vi "ReadGatewayConfigurationFile.vi"(8 "error in (no error)":errorcluster, 11 "targets.ini file":path) -> (0 "error out":errorcluster, 3 "Gateway Configuration":T1)   [LabVIEW 2024, in "VeriStandTestUtilities.lvlib"]
uses:
  VeriStandTestUtilities.lvlib
  GatewayConfiguration.ctl
  <vilib>/Utility/config.llb/Read Key (String).vi
  <vilib>/Utility/config.llb/NI_LVConfig.lvlib
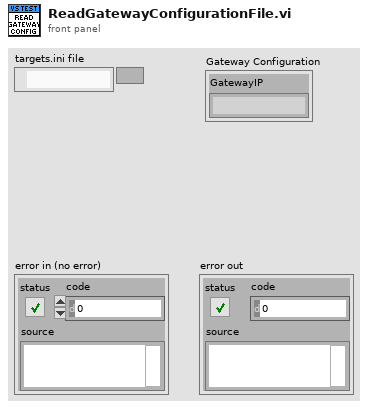
[diagram p1: front panel]
types:
  T1 = typedef "VeriStandTestUtilities.lvlib/GatewayConfiguration.ctl" = cluster{"GatewayIP":string}
  T2 = typedef "NI_LVConfig.lvlib/Config Data RefNum.ctl" = refnum<k1>
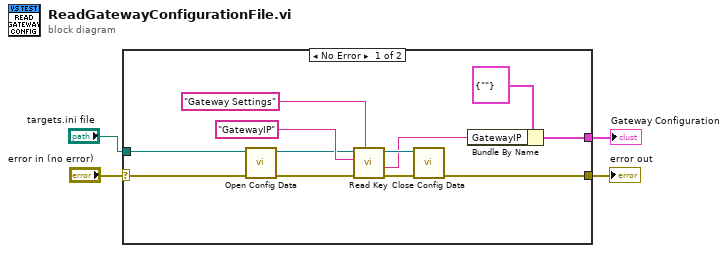
[diagram p0: block diagram]
diagram:
  n1 = case shown="No Error" "error in (no error)" {
    selector: "error in (no error)" -> [w15 w17]
    tunnel: [w6 w17] -> w3
    tunnel: "targets.ini file" -> [w16 _]
    tunnel: [w10 _] -> w1
    frame No Error {
      n2 = call <vilib>:"Open Config Data.vi"("error in (no error)"=w15, "configuration file path"=w16) -> ("error out"=w8:errorcluster, "refnum"=w9:T2)  [unwired: 7 in, 1 out]
      n3 = call-poly <vilib>:"Read Key.vi"("section"="Gateway Settings", "error in (no error)"=w8, "key"="GatewayIP", "refnum"=w9) -> ("error out"=w14:errorcluster, "value"=w5:string, "refnum out"=w13:T2)  [unwired: 4 in, 1 out]
      n4 = call <vilib>:"Close Config Data.vi"("error in (no error)"=w14, "refnum"=w13) -> ("error out"=w6:errorcluster)  [unwired: 8 in, 1 out]
      n5 = Bundle By Name(cluster=T1 {"GatewayIP"=""} ("Gateway Configuration"), "GatewayIP"=w5) -> (w10:T1)
    }
    frame Error {
    }
  }
  "error out" <- w3
  "Gateway Configuration" <- w1
